vi "Gas_Release_Control.vi"(5 "Extra Commands":string, 6 "Density Ratio":string="Carrier 1 only", 7 "Strength (% by volume)":dbl format="%.3f", 8 "Stack flowrate (l/min)":dbl format="%.2f", 9 "Source Status":T2) -> (0 "error out":errorcluster, 1 "Flowrates (kg/min)":dbl[](array[numeric]) format="%.2f", 2 "Source Est Time (s)":dbl, 3 "Flowrates Achieved?":bool)   [LabVIEW 2012]
uses:
  ADAM Controls/Client_Source_Status.ctl
  ADAM Controls/Client_Source.ctl
  ADAM Controls/Channel_names.ctl
  ADAM Controls/Module_type_ADAM.ctl
  ADAM Controls/Calib_type_ADAM.ctl
  ADAM Controls/Channel_State.ctl
  ADAM Controls/Ch_description_ADAM.ctl
  ADAM Controls/Function_ADAM.ctl
  ADAM Controls/Address.ctl
  ADAM Controls/Update_scan_value.ctl
  Anemometry/Anemometry Sub Vis/Controls/In_Range.ctl
  Anemometry/Anemometry Sub Vis/Globals/Preference_global.vi
  Anemometry/Anemometry Sub Vis/Globals/Extra_Commands_Global.vi
panel:
  out "Error String":string
  out "Currently on":T1=enum."Get Source Clients"
  out "Status of other Clients":string[](array[string])
  out "Source already correct?":bool
  out "No Other Clients are Using Source?":bool
  out "Source Clients":string[](array[string])
  # "-Carrier 1 only\n-Carrier 2 only\n-Enter Ratio"
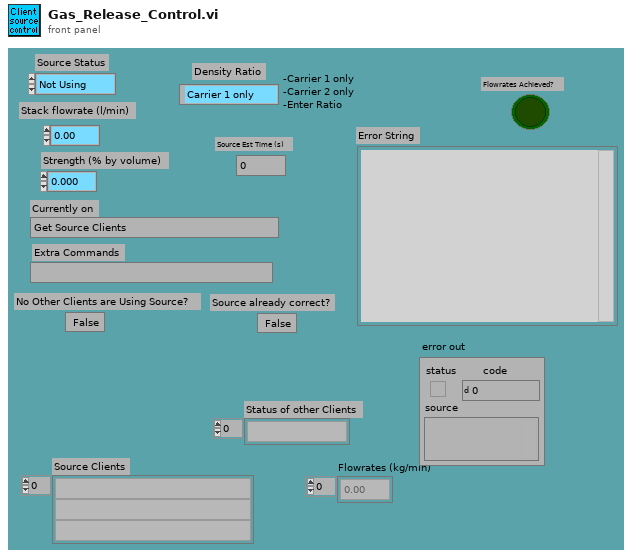
[diagram p1: front panel]
types:
  T1 = typedef "Client_Source.ctl" = enum16{"Start", "Get Source Clients", "Has this client liberty to control the source?", "Declare not using, other client already waiting", "Is the Source already correct?", "Declare waiting, other client is still using", "Control Hi-Tec", "Were the Hi-tecs able to achieve the flowrates?", "Declare source status", "Wait for source to Establish"}
  T2 = typedef "Client_Source_Status.ctl" = enum16{"Not Using", "Using", "Must Have"}
  T3 = typedef "Channel_names.ctl" = enum16{"Active Only", "Active + Off", "All Channels"}
  T4 = typedef "Ch_description_ADAM.ctl" = cluster{"Ch Name":string, "Type":T5, "Function":T6, "Ch State":T7, "Calibration type":T8, "A":dbl, "B":dbl, "C":dbl, "D":dbl, "Comments":string, "Address":T9, "String":string, "Duty":u16}
  T5 = typedef "Module_type_ADAM.ctl" = string
  T6 = typedef "Function_ADAM.ctl" = enum16{"Analogue Input", "Digital Input", "Event counter", "Event rate", "Analogue Output", "Digital Output", "Relay Output"}
  T7 = typedef "Channel_State.ctl" = enum16{"On", "Off", "Always On", "Always Off"}
  T8 = typedef "Calib_type_ADAM.ctl" = enum16{"Raw", "Bx + A", "Cx^2 + Bx + A", "Dx^3 + Cx^2 + Bx + A", "In Band", "Hi-Tec Q", "Hi-Tec M_dot", "Text"}
  T9 = typedef "Address.ctl" = cluster{"Main":i32, "Ch.":i32, "Sub":i32, "Port Name":string}
  T10 = typedef "Update_scan_value.ctl" = cluster{"Channel Name":string, "New Value":dbl}
  T11 = typedef "In_Range.ctl" = enum16{"%", "±", "% & ±"}
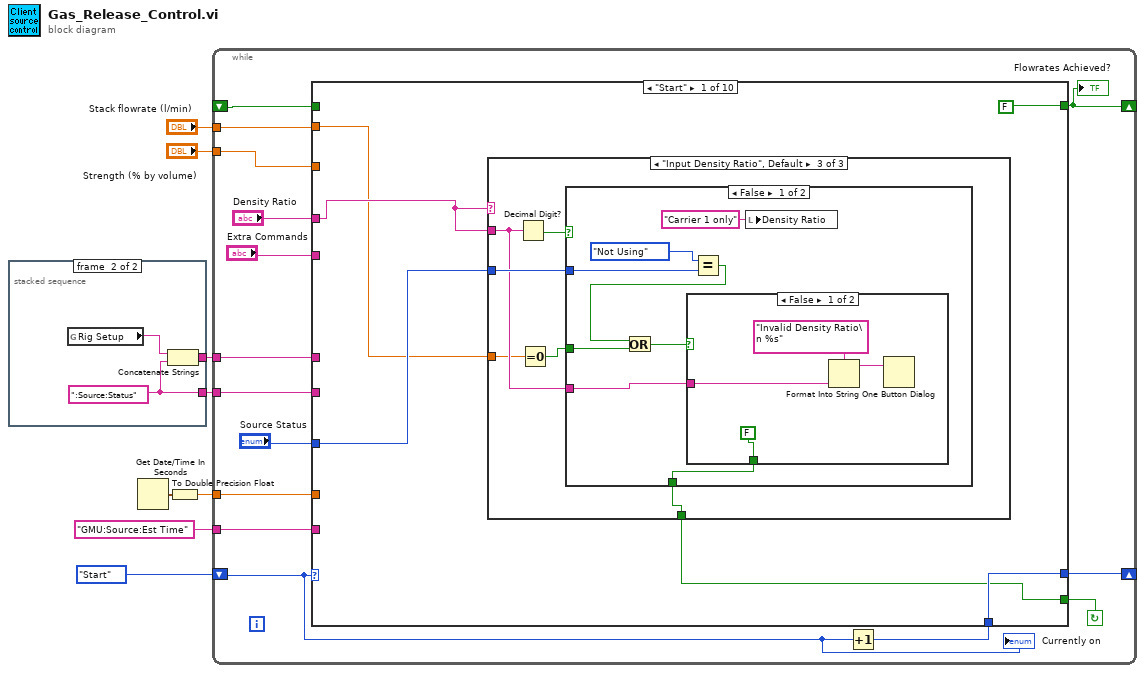
[diagram p0: block diagram]
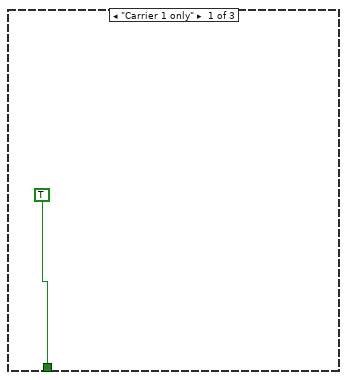
[diagram p2: hidden frame]
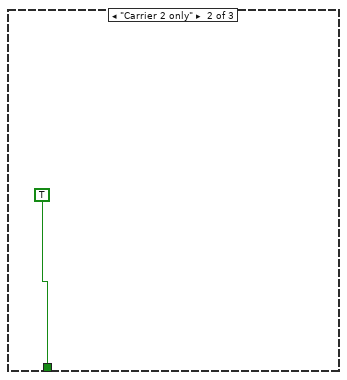
[diagram p3: hidden frame]
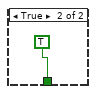
[diagram p4: hidden frame]
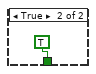
[diagram p5: hidden frame]
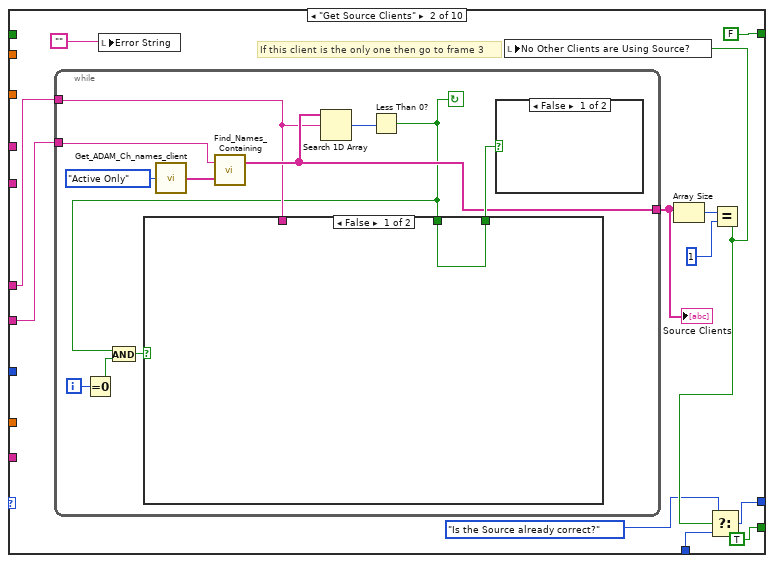
[diagram p6: hidden frame]
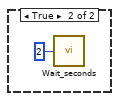
[diagram p7: hidden frame]
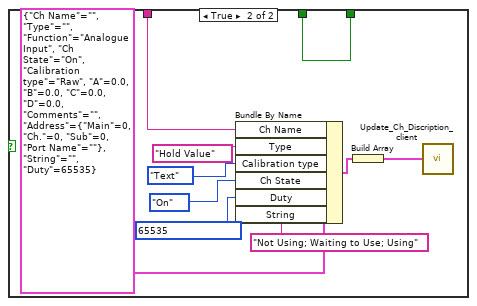
[diagram p8: hidden frame]
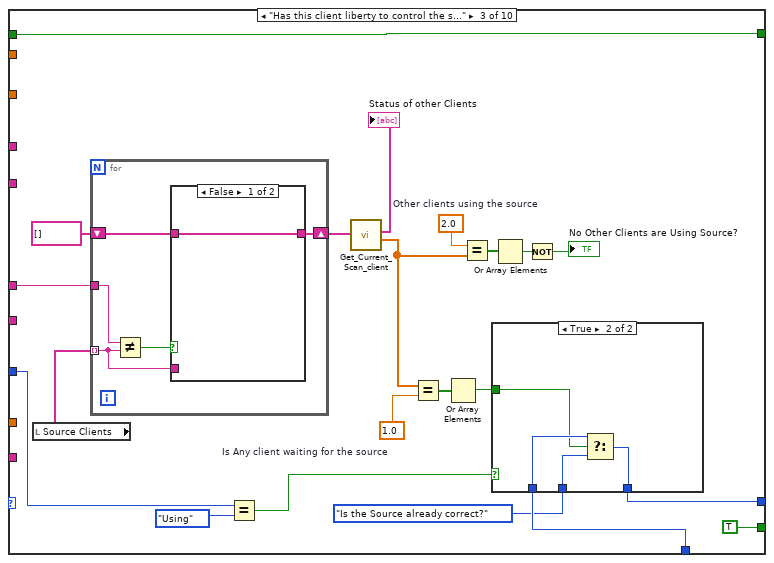
[diagram p9: hidden frame]
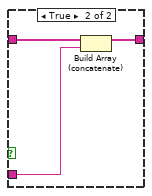
[diagram p11: hidden frame]
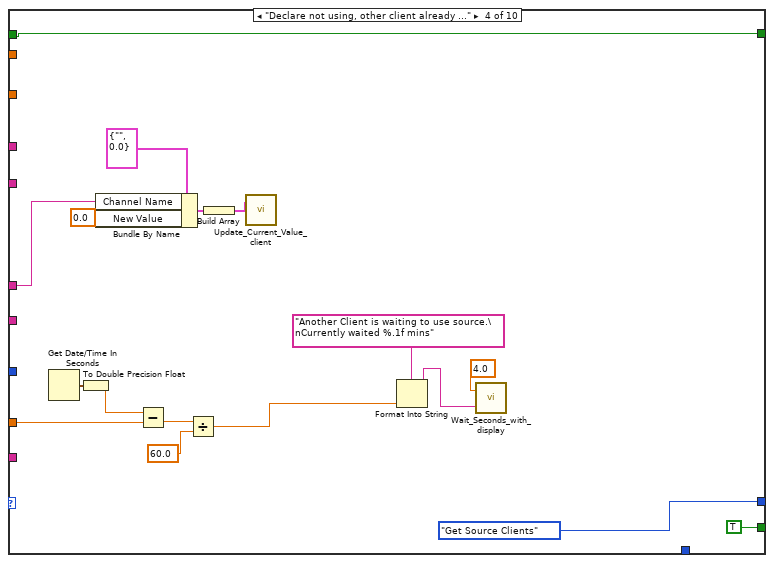
[diagram p12: hidden frame]
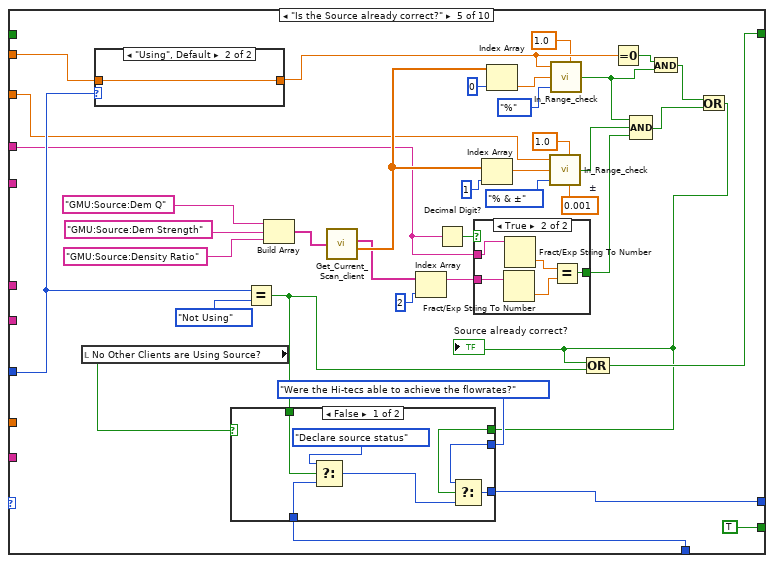
[diagram p13: hidden frame]
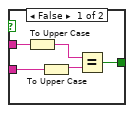
[diagram p14: hidden frame]
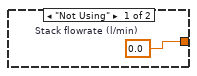
[diagram p15: hidden frame]
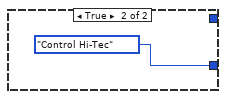
[diagram p16: hidden frame]
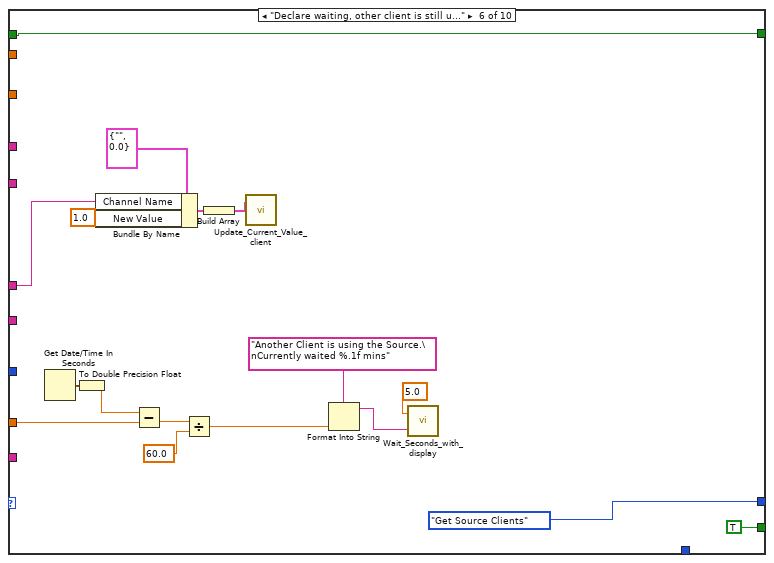
[diagram p17: hidden frame]
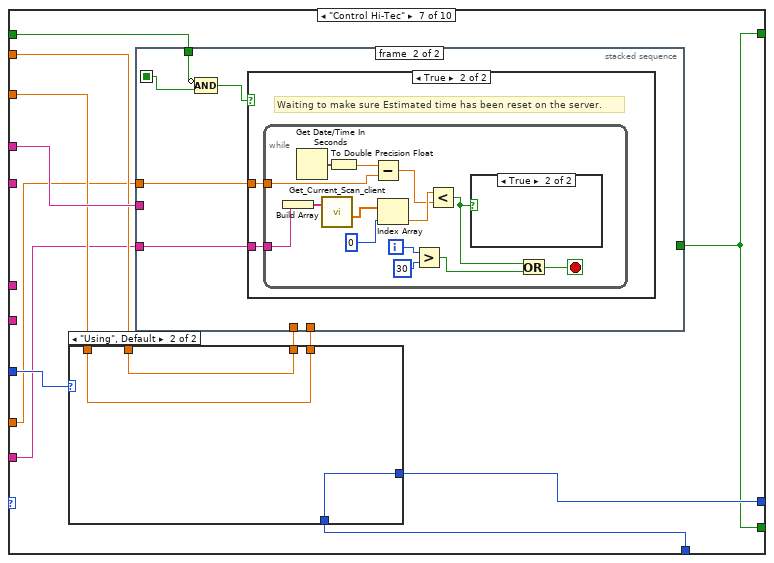
[diagram p18: hidden frame]
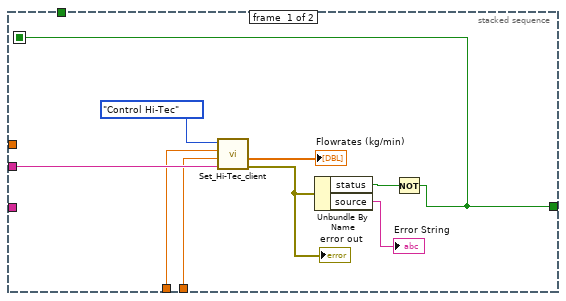
[diagram p19: hidden frame]
diagram:
  n1 = stacked-sequence {
    tunnel: [_ w11] -> w8
    tunnel: [_ w10] -> w7
    frame #0 {
      n2 = call "Run_EnFlo_Hub.vi"() -> ()  [unwired: 8 out]
    }
    frame #1 {
      w11 = ":Source:Status"
      n3 = global read "Preference_global.vi" "Rig Setup"() -> (w9:string)
      n4 = Concatenate Strings(w9, w11) -> (w10:string)
    }
  }
  n5 = Get Date/Time In Seconds() -> (seconds since 1Jan1904=w2:timestamp)
  n6 = To Double Precision Float(number=w2) -> (double precision float=w6:dbl)
  n7 = while {
    tunnel: w6 -> [w22]
    tunnel: w7 -> [w25]
    shift-left: Client_Source."Start" -> [w20]
    shift-right: [w21] -> _
    tunnel: w8 -> [w26]
    tunnel: "Stack flowrate (l/min)" -> [w16]
    tunnel: "Strength (% by volume)" -> [w15]
    shift-right: [w13] -> _
    shift-left: _ -> [w14]
    tunnel: "GMU:Source:Est Time" -> [w12]
    stop <- w24 continue-if-true
    n8 = Increment(x=w20) -> (x+1=w23:T1)
    n9 = case shown="\"Start\"" w20 {
      tunnel: w16 -> [w27 _ _ _ w172 _ w225 w270 _ w318]
      tunnel: w15 -> [_ _ _ _ w155 _ w223 _ _ _]
      tunnel: "Density Ratio" -> [w31 _ _ _ w147 _ w228 _ _ _]
      tunnel: w26 -> [_ w66 _ _ _ _ _ _ _ _]
      tunnel: [w32 w62 w103 Client_Source."Get Source Clients" w143 Client_Source."Get Source Clients" w222 w272 w308 w324] -> w21
      tunnel: w25 -> [_ w65 w110 w136 _ w211 _ _ w314 _]
      tunnel: [w30 TRUE TRUE TRUE TRUE TRUE w218 TRUE TRUE FALSE] -> w24
      tunnel: w23 -> [w32 w61 w105 _ w173 _ w221 w271 w308 w324]
      tunnel: w22 -> [_ _ _ w134 _ w206 w219 _ _ _]
      tunnel: "Source Status" -> [w29 _ w94 _ w164 _ w227 w269 w312 w323]
      tunnel: "Extra Commands" -> [_ _ _ _ _ _ _ _ _ w321]
      tunnel: [FALSE FALSE w90 w126 w145 w201 w218 w268 w306 w319] -> w13
      tunnel: w14 -> [_ _ w90 w126 _ w201 w217 _ w306 w319]
      tunnel: w12 -> [_ _ _ _ _ _ w220 w266 _ _]
      frame "Start" {
        n10 = case shown="\"Input Density Ratio\", Default" w31 {
          tunnel: w31 -> [_ _ w37]
          tunnel: [TRUE TRUE w38] -> w30
          tunnel: w29 -> [_ _ w39]
          tunnel: w27 -> [_ _ w36]
          frame "Carrier 1 only" {
            (unwired) TRUE
            (unwired) 0.0 ("Qc2")
          }
          frame "Carrier 2 only" {
            (unwired) TRUE
            (unwired) 0.0 ("Qc1")
          }
          frame "Input Density Ratio", Default {
            n11 = Decimal Digit?(1:w37) -> (0:w40:bool)
            n12 = Equal To 0?(x=w36) -> (x = 0?=w35:bool)
            n13 = case shown="False" w40 {
              tunnel: w39 -> [w47 _]
              tunnel: [w46 TRUE] -> w38
              tunnel: w37 -> [w45 _]
              tunnel: w35 -> [w42 _]
              frame False {
                n14 = Equal?(x=Client_Source_Status."Not Using" ("Source Status"), y=w47) -> (x = y?=w43:bool)
                n15 = Or(x=w43, y=w42) -> (x .or. y?=w41:bool)
                n16 = case shown="False" w41 {
                  tunnel: [FALSE TRUE] -> w46
                  tunnel: w45 -> [w52 _]
                  frame False {
                    n17 = Format Into String(format string="Invalid Density Ratio\n %s", w52) -> (resulting string=w50:string)  [unwired: 2 in, 1 out]
                    n18 = One Button Dialog(message=w50) -> ()  [unwired: 2 out]
                  }
                  frame True {
                  }
                }
                n19 = local write "Density Ratio"("Carrier 1 only" ("Density Ratio")) -> ()
              }
              frame True {
              }
            }
          }
        }
      }
      frame "Get Source Clients" {
        # "If this client is the only one then go to frame 3"
        n20 = while {
          tunnel: [w70] -> w59
          tunnel: w65 -> [w69]
          tunnel: w66 -> [w77]
          i -> [w74]
          stop <- w67 continue-if-true
          n21 = Equal To 0?(x=w74) -> (x = 0?=w73:bool)
          n22 = call "Get_ADAM_Ch_names_client.vi"("Channel names set"=Channel_names."Active Only") -> ("Ch names"=w75:string[])
          n23 = call "Find_Names_Containing.vi"("Ch names"=w75, "String to match"=w77) -> ("Matched Names"=w70:string[])  [unwired: 1 out]
          n24 = Search 1D Array(1D array=w70, element=w69) -> (index of element=w68:i32)  [unwired: 1 out]
          n25 = Less Than 0?(x=w68) -> (x < 0?=w67:bool)
          n26 = And(x=w67, y=w73) -> (x .and. y?=w72:bool)
          n27 = case shown="False" w72 {
            tunnel: w69 -> [_ w86]
            tunnel: [w79 w82] -> w71
            tunnel: w67 -> [w79 w82]
            frame False {
            }
            frame True {
              n28 = Bundle By Name(cluster=T4 {"Ch Name"="", "Type"="", "Function"=enum."Analogue Input", "Ch State"=enum."On", "Calibration type"=enum."Raw", "A"=0.0, "B"=0.0, "C"=0.0, "D"=0.0, "Comments"="", "Address"={"Main"=0, "Ch."=0, "Sub"=0, "Port Name"=""}, "String"="", "Duty"=65535} ("Ch Discription"), "Ch Name"=w86, "Type"=T5 "Hold Value", "Calibration type"=Calib_type_ADAM."Text", "Ch State"=Channel_State."On", "Duty"=u16 65535 ("Bundle Element"), "String"="Not Using; Waiting to Use; Using") -> (w84:T4)
              n29 = Build Array(w84) -> (w83:T4[])
              n30 = call "Update_Ch_Discription_client.vi"("Channels to update In"=w83) -> ()  [unwired: 1 out]
            }
          }
          n31 = case shown="False" w71 {
            frame False {
            }
            frame True {
              n32 = call "Wait_seconds.vi"("Seconds to wait"=u32 2) -> ()
            }
          }
        }
        "Source Clients" <- w59
        n33 = local write "Error String"("") -> ()
        n34 = Array Size(array=w59) -> (size(s)=w64:i32)
        n35 = Equal?(x=w64, y=1) -> (x = y?=w58:bool)
        n36 = local write "No Other Clients are Using Source?"(w58) -> ()
        n37 = Select(t=Client_Source."Is the Source already correct?", s=w58, f=w61) -> (s? t:f=w62:T1)
      }
      frame "Has this client liberty to control the source?" {
        w102 = 2.0  # Other clients using the source
        w108 = 1.0  # Is Any client waiting for the source
        n38 = local read "Source Clients"() -> (w104:string[])
        n39 = for {
          tunnel: w104 -> [w116] mode=indexing
          tunnel: w110 -> [w120]
          shift-right: [w117] -> w100
          shift-left: string[] [] -> [w118]
          n40 = Not Equal?(x=w120, y=w116) -> (x != y?=w119:bool)
          n41 = case shown="False" w119 {
            tunnel: w118 -> [w121 w124]
            tunnel: [w121 w123] -> w117
            tunnel: w116 -> [_ w122]
            frame False {
            }
            frame True {
              n42 = Build Array (concatenate)(w124, w122) -> (w123:string[])
            }
          }
        }
        n43 = Equal?(x=w94, y=Client_Source_Status."Using" ("Source Status")) -> (x = y?=w93:bool)
        n44 = call "Get_Current_Scan_client.vi"("ADAM Ch Names"=w100) -> ("String values"=→"Status of other Clients":string[], "Numerical Values"=w97:dbl[])  [unwired: 2 out]
        n45 = Equal?(x=w97, y=w108) -> (x = y?=w107:bool[])
        n46 = Or Array Elements(Boolean array=w107) -> (logical OR=w98:bool)
        n47 = Equal?(x=w102, y=w97) -> (x = y?=w101:bool[])
        n48 = case shown="True" w93 {
          tunnel: w105 -> [_ w115]
          tunnel: [w111 w114] -> w103
          tunnel: w98 -> [_ w113]
          tunnel: Client_Source."Is the Source already correct?" -> [w111 w112]
          frame False {
          }
          frame True {
            n49 = Select(t=w115, s=w113, f=w112) -> (s? t:f=w114:T1)
          }
        }
        n50 = Or Array Elements(Boolean array=w101) -> (logical OR=w96:bool)
        n51 = Not(x=w96) -> (.not. x?=→"No Other Clients are Using Source?":bool)
      }
      frame "Declare not using, other client already waiting" {
        n52 = Get Date/Time In Seconds() -> (seconds since 1Jan1904=w125:timestamp)
        n53 = To Double Precision Float(number=w125) -> (double precision float=w135:dbl)
        n54 = Bundle By Name(cluster=T10 {"Channel Name"="", "New Value"=0.0} ("Update Scan Value Cluster"), "Channel Name"=w136, "New Value"=0.0 ("Bundle Element")) -> (w139:T10)
        n55 = Subtract(x=w135, y=w134) -> (x-y=w133:dbl)
        n56 = Divide(x=w133, y=60.0) -> (x/y=w127:dbl)
        n57 = Build Array(w139) -> (w138:T10[])
        n58 = call "Update_Current_Value_client.vi"("Update array in"=w138) -> ()  [unwired: 1 in]
        n59 = Format Into String(format string="Another Client is waiting to use source.\nCurrently waited %.1f mins" ("Format String"), w127) -> (resulting string=w130:string)  [unwired: 2 in, 1 out]
        n60 = call "Wait_Seconds_with_display.vi"("Message"=w130, "Seconds to wait"=4.0) -> ()  [unwired: 2 out]
      }
      frame "Is the Source already correct?" {
        w152 = 0.001  # ±
        n61 = local read "No Other Clients are Using Source?"() -> (w174:bool)
        n62 = case shown="\"Using\", Default" w164 {
          tunnel: [w190 w191] -> w162
          tunnel: w172 -> [_ w191]
          frame "Not Using" {
            w190 = 0.0  # Stack flowrate (l/min)
          }
          frame "Using", Default {
          }
        }
        n63 = Equal?(x=w164, y=Client_Source_Status."Not Using" ("Source Status")) -> (x = y?=w163:bool)
        n64 = Build Array("GMU:Source:Dem Q", "GMU:Source:Dem Strength", "GMU:Source:Density Ratio") -> (w176:string[])
        n65 = call "Get_Current_Scan_client.vi"("ADAM Ch Names"=w176) -> ("String values"=w149:string[], "Numerical Values"=w169:dbl[])  [unwired: 2 out]
        n66 = Index Array(array=w149, index=2 ("Index")) -> (element=w148:string)
        n67 = Decimal Digit?(1:w147) -> (0:w151:bool)
        n68 = case shown="True" w151 {
          tunnel: [w183 w186] -> w146
          tunnel: w147 -> [w182 w188]
          tunnel: w148 -> [w181 w189]
          frame False {
            n69 = To Upper Case(1:w182) -> (0:w184:string)
            n70 = To Upper Case(1:w181) -> (0:w180:string)
            n71 = Equal?(x=w184, y=w180) -> (x = y?=w183:bool)
          }
          frame True {
            n72 = Fract/Exp String To Number(string=w189) -> (number=w185:dbl)  [unwired: 4 out]
            n73 = Fract/Exp String To Number(string=w188) -> (number=w187:dbl)  [unwired: 4 out]
            n74 = Equal?(x=w187, y=w185) -> (x = y?=w186:bool)
          }
        }
        n75 = Index Array(array=w169, index=1 ("Index")) -> (element=w154:dbl)
        n76 = Index Array(array=w169, index=0 ("Index")) -> (element=w161:dbl)
        n77 = call "In_Range_check.vi"("±"=w152, "%"=1.0, "Mode"=In_Range."% & ±", "Value"=w154, "Setpoint"=w155) -> ("In Range"=w153:bool)  [unwired: 2 out]
        n78 = call "In_Range_check.vi"("%"=1.0, "Mode"=In_Range."%", "Value"=w161, "Setpoint"=w162) -> ("In Range"=w160:bool)  [unwired: 1 in, 2 out]
        n79 = Equal To 0?(x=w162) -> (x = 0?=w168:bool)
        n80 = Compound Arithmetic op=AND(w160, w153, w146) -> (w166:bool)
        n81 = And(x=w168, y=w160) -> (x .and. y?=w167:bool)
        n82 = Or(x=w167, y=w166) -> (x .or. y?=w142:bool)
        "Source already correct?" <- w142
        n83 = case shown="False" w174 {
          tunnel: w173 -> [w198 _]
          tunnel: w163 -> [w197 _]
          tunnel: w142 -> [w195 _]
          tunnel: Client_Source."Were the Hi-tecs able to achieve the flowrates?" -> [w193 _]
          tunnel: [w192 Client_Source."Control Hi-Tec"] -> w143
          frame False {
            n84 = Select(t=Client_Source."Declare source status", s=w197, f=w198) -> (s? t:f=w194:T1)
            n85 = Select(t=w193, s=w195, f=w194) -> (s? t:f=w192:T1)
          }
          frame True {
          }
        }
        n86 = Compound Arithmetic op=OR(w142, w163) -> (w145:bool)
      }
      frame "Declare waiting, other client is still using" {
        n87 = Get Date/Time In Seconds() -> (seconds since 1Jan1904=w200:timestamp)
        n88 = To Double Precision Float(number=w200) -> (double precision float=w209:dbl)
        n89 = Bundle By Name(cluster=T10 {"Channel Name"="", "New Value"=0.0} ("Update Scan Value Cluster"), "Channel Name"=w211, "New Value"=1.0 ("Bundle Element")) -> (w214:T10)
        n90 = Subtract(x=w209, y=w206) -> (x-y=w208:dbl)
        n91 = Divide(x=w208, y=60.0) -> (x/y=w202:dbl)
        n92 = Build Array(w214) -> (w213:T10[])
        n93 = call "Update_Current_Value_client.vi"("Update array in"=w213) -> ()  [unwired: 1 in]
        n94 = Format Into String(format string="Another Client is using the Source.\nCurrently waited %.1f mins" ("Format String"), w202) -> (resulting string=w205:string)  [unwired: 2 in, 1 out]
        n95 = call "Wait_Seconds_with_display.vi"("Message"=w205, "Seconds to wait"=5.0) -> ()  [unwired: 2 out]
      }
      frame "Control Hi-Tec" {
        n96 = case shown="\"Using\", Default" w227 {
          tunnel: [w262 w265] -> w226
          tunnel: w225 -> [_ w265]
          tunnel: [w261 w264] -> w224
          tunnel: w223 -> [_ w264]
          tunnel: [Client_Source."Declare source status" w263] -> w222
          tunnel: w221 -> [_ w263]
          frame "Not Using" {
            w261 = 0.0  # Strength (% by volume)
            w262 = 0.0  # Stack flowrate (l/min)
          }
          frame "Using", Default {
          }
        }
        n97 = stacked-sequence {
          seq-local: [w229 _] -> [_ w240]
          tunnel: w228 -> [w236 _]
          tunnel: w226 -> [w234 _]
          tunnel: w224 -> [w233 _]
          tunnel: w220 -> [_ w242]
          tunnel: w219 -> [_ w241]
          tunnel: [w229 _] -> w218
          tunnel: w217 -> [_ w239]
          frame #0 {
            n98 = call "Set_Hi-Tec_client.vi"("Density Ratio"=w236, "Strength (% by volume)"=w233, "Stack flowrate (l/min)"=w234, "Mode"=enum16{"Control Hi-Tec", "Check Hi-Tec Demands"}."Control Hi-Tec") -> ("error out"=w232:errorcluster, "Flowrates (kg/min)"=→"Flowrates (kg/min)":dbl[])  [unwired: 1 in, 3 out]
            "error out" <- w232
            n99 = Unbundle By Name(w232) -> ("status"=w230:bool, "source"=→"Error String":string)
            n100 = Not(x=w230) -> (.not. x?=w229:bool)
          }
          frame #1 {
            n101 = Compound Arithmetic op=AND(invert w239, w240) -> (w238:bool)
            n102 = case shown="True" w238 {
              tunnel: w242 -> [_ w244]
              tunnel: w241 -> [_ w243]
              frame False {
              }
              frame True {
                # "Waiting to make sure Estimated time has been reset on the server."
                n103 = while {
                  tunnel: w244 -> [w257]
                  tunnel: w243 -> [w252]
                  i -> [w249]
                  stop <- w245 stop-if-true
                  n104 = Build Array(w257) -> (w258:string[])
                  n105 = Get Date/Time In Seconds() -> (seconds since 1Jan1904=w254:timestamp)
                  n106 = call "Get_Current_Scan_client.vi"("ADAM Ch Names"=w258) -> ("Numerical Values"=w256:dbl[])  [unwired: 3 out]
                  n107 = To Double Precision Float(number=w254) -> (double precision float=w253:dbl)
                  n108 = Subtract(x=w253, y=w252) -> (x-y=w250:dbl)
                  n109 = Index Array(array=w256, index=0) -> (element=w251:dbl)
                  n110 = Greater?(x=w249, y=30) -> (0:w246:bool)
                  n111 = Less?(x=w251, y=w250) -> (x < y?=w247:bool)
                  n112 = case shown="True" w247 {
                    frame False {
                      n113 = Wait (ms)(milliseconds to wait=u32 1000) -> ()  [unwired: 1 out]
                    }
                    frame True {
                    }
                  }
                  n114 = Or(x=w247, y=w246) -> (x .or. y?=w245:bool)
                }
              }
            }
          }
        }
      }
      frame "Were the Hi-tecs able to achieve the flowrates?" {
        n115 = Get Date/Time In Seconds() -> (seconds since 1Jan1904=w267:timestamp)
        n116 = To Double Precision Float(number=w267) -> (double precision float=w274:dbl)
        n117 = while {
          tunnel: w269 -> [w282]
          tunnel: w270 -> [w280]
          tunnel: [w278] -> w273
          tunnel: w274 -> [w295]
          tunnel: [w278] -> w268
          tunnel: w266 -> [w276]
          stop <- w291 continue-if-true
          w279 = 0.1  # ±
          w287 = 1.0  # %
          n118 = case shown="\"Using\", Default" w282 {
            tunnel: [w300 w301] -> w281
            tunnel: w280 -> [_ w301]
            frame "Not Using" {
              w300 = 0.0  # Stack flowrate (l/min)
            }
            frame "Using", Default {
            }
          }
          n119 = Get Date/Time In Seconds() -> (seconds since 1Jan1904=w277:timestamp)
          n120 = To Double Precision Float(number=w277) -> (double precision float=w296:dbl)
          n121 = Subtract(x=w296, y=w295) -> (x-y=w294:dbl)
          n122 = Build Array("GMU:Source:Dem Q", w276) -> (w299:string[])
          n123 = Less?(x=w294, y=120.0) -> (x < y?=w292:bool)
          n124 = call "Get_Current_Scan_client.vi"("ADAM Ch Names"=w299) -> ("Numerical Values"=w285:dbl[])  [unwired: 3 out]
          n125 = Index Array(array=w285, index=1 ("Index")) -> (element=w297:dbl)
          "Source Est Time (s)" <- w297
          n126 = Index Array(array=w285, index=0 ("Index")) -> (element=w289:dbl)
          n127 = Greater Than 0?(x=w297) -> (x > 0?=w283:bool)
          n128 = call "In_Range_check.vi"("±"=w279, "%"=w287, "Mode"=In_Range."% & ±", "Value"=w289, "Setpoint"=w281) -> ("In Range"=w284:bool)  [unwired: 2 out]
          n129 = And(x=w284, y=w283) -> (x .and. y?=w278:bool)
          n130 = Compound Arithmetic op=AND(invert w278, w292) -> (w291:bool)
          n131 = case shown="True" w291 {
            frame False {
            }
            frame True {
              n132 = Wait (ms)(milliseconds to wait=u32 1000) -> ()  [unwired: 1 out]
            }
          }
        }
        n133 = case shown="True" w273 {
          tunnel: [Client_Source."Control Hi-Tec" w305] -> w272
          tunnel: w271 -> [_ w305]
          frame False {
            n134 = local write "Source Status"(Client_Source_Status."Not Using" ("Source Status")) -> ()
          }
          frame True {
          }
        }
      }
      frame "Declare source status" {
        n135 = case shown="\"Using\"" w312 {
          tunnel: [0.0 2.0 2.0] -> w307
          frame "Not Using" {
          }
          frame "Using" {
          }
          frame "Must Have" {
          }
        }
        n136 = Bundle By Name(cluster=T10 {"Channel Name"="", "New Value"=0.0} ("Update Scan Value Cluster"), "Channel Name"=w314, "New Value"=w307) -> (w310:T10)
        n137 = Build Array(w310) -> (w309:T10[])
        n138 = call "Update_Current_Value_client.vi"("Update array in"=w309) -> ()  [unwired: 1 in]
      }
      frame "Wait for source to Establish" {
        n139 = Not Equal?(x=Client_Source_Status."Not Using" ("Source Status"), y=w323) -> (x != y?=w320:bool)
        n140 = case shown="True" w320 {
          tunnel: w321 -> [_ w342]
          tunnel: w318 -> [_ w331]
          frame False {
          }
          frame True {
            n141 = global read "Extra_Commands_Global.vi" "Establish Exp Conditions (s)"() -> (w343:string)
            n142 = global read "Preference_global.vi" "Default Source Establishment Time (s)"() -> (w334:dbl)
            n143 = Equal To 0?(x=w331) -> (x = 0?=w329:bool)
            n144 = Divide(x=100.0, y=w331) -> (x/y=w328:dbl)
            n145 = local read "Source Est Time (s)"() -> (w335:dbl)
            n146 = Not A Number/Path/Refnum?(number/path/refnum=w335) -> (NaN/Path/Refnum?=w339:bool)
            n147 = call "Extra_Commands.vi"("String to Search"=w342, "Command"=w343) -> ("Numeric Value"=w336:dbl, "Command Found"=w337:bool)  [unwired: 1 in, 3 out]
            n148 = Select(t=w336, s=w337, f=w334) -> (s? t:f=w333:dbl)
            n149 = Select(t=0.0, s=w329, f=w328) -> (s? t:f=w326:dbl)
            n150 = Add(x=w326, y=w333) -> (x+y=w332:dbl)
            n151 = Subtract(x=w332, y=w335) -> (x-y=w338:dbl)
            n152 = Greater Than 0?(x=w338) -> (x > 0?=w341:bool)
            n153 = Or(x=w341, y=w339) -> (x .or. y?=w340:bool)
            n154 = case shown="True" w340 {
              tunnel: w339 -> [_ w347]
              tunnel: w332 -> [_ w346]
              tunnel: w338 -> [_ w345]
              frame False {
              }
              frame True {
                n155 = Select(t=w346, s=w347, f=w345) -> (s? t:f=w344:dbl)
                n156 = call "Wait_Seconds_with_display.vi"("Message"="Establishing Source", "Seconds to wait"=w344) -> ()  [unwired: 2 out]
              }
            }
          }
        }
      }
    }
    "Flowrates Achieved?" <- w13
    "Currently on" <- w20
  }
